vi "Init Device.vi"(8 "error in (no error)":errorcluster, 11 "Toggle 6 in":refnum<class "Toggle 6.lvclass">) -> (0 "error out":errorcluster, 3 "Toggle 6 out":refnum<class "Toggle 6.lvclass">)   [LabVIEW 2020, in "Toggle 6.lvclass"]
doc: "Init the device and writes all default values into registers"
uses:
  Toggle 6.lvclass
  PIC-device/PIC-Device.lvclass
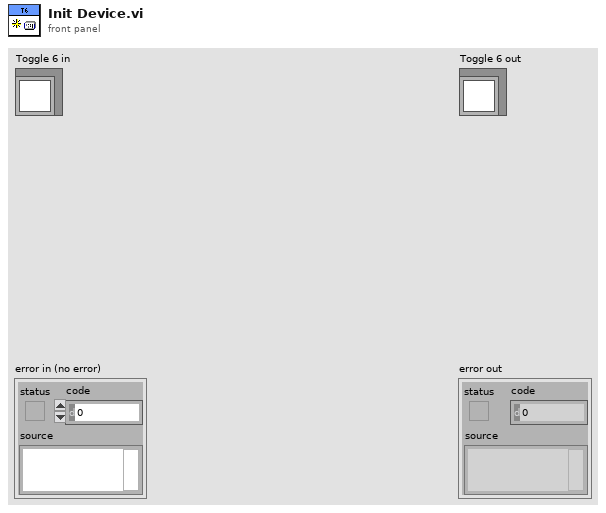
[diagram p1: front panel]
types:
  T1 = enum16{"RFFE 2-wire", "WiSPI 3-wire spi_sel", "WiSPI 4-wire spi_sel", "ifxSPI 3-wire spi_sel", "WiSPI 3-wire dev add spi_sel"}
  T2 = typedef "PIC-Device.lvclass/Register to Write.ctl" = cluster{"Register":u32, "Value":u32, "Dev Address":u32, "Physical Adress":u32}
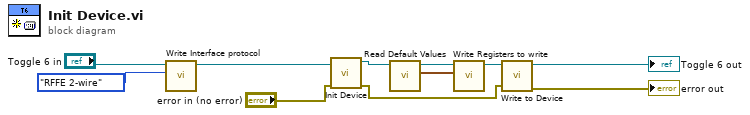
[diagram p0: block diagram]
diagram:
  n1 = call-dynamic "Write Interface protocol.vi"("Interface protocol"=T1."RFFE 2-wire", "Device in"="Toggle 6 in") -> ("Device out"=w10:refnum<class "Toggle 6.lvclass">)  [unwired: 9 in]
  n2 = call-parent "Init Device.vi"("error in (no error)"="error in (no error)", "Device in"=w10) -> ("error out"=w3:errorcluster, "Device out"=w7:refnum<class "Toggle 6.lvclass">)  [unwired: 8 in]
  n3 = call-dynamic "Read Default Values.vi"("Toggle 6 in"=w7) -> ("Default Values"=w5:T2[], "Toggle 6 out"=w6:refnum<class "Toggle 6.lvclass">)  [unwired: 9 in]
  n4 = call-dynamic "Write Registers to write.vi"("Registers to write"=w5, "Device in"=w6) -> ("Device out"=w4:refnum<class "Toggle 6.lvclass">)  [unwired: 9 in]
  n5 = call-dynamic "Write to Device.vi"("error in (no error)"=w3, "Device in"=w4) -> ("error out"=→"error out":errorcluster, "Device out"=→"Toggle 6 out":refnum<class "Toggle 6.lvclass">)  [unwired: 7 in, 1 out]
